vi "Graph_Input_v00.vi"(11 "Control":T7={"PII In 1"={"Lock"=FALSE, "Hold"=FALSE, "P Gain"=0, "P BS"=-5, "I Gain"=0, "I BS"=-10, "I2 G"=0, "I2 BS"=-26, "Scan Amp"=0, "Scan Off"=0, "Scan FS"=0, "SFS BS"=0, "I Max value"=10000, "I2 Max value"=10000, "Scope.Offset"=0, "Trigger Direction"=enum."either", "Scan-PII thresh"=0}, "PII In 2"={"Lock"=FALSE, "Hold"=FALSE, "P Gain"=0, "P BS"=-10, "I Gain"=0, "I BS"=-10, "I2 G"=0, "I2 BS"=-26, "Scan Amp"=0, "Scan Off"=0, "Scan FS"=0, "SFS BS"=0, "I Max value"=10000, "I2 Max value"=10000, "Scope.Offset"=0, "Trigger Direction"=enum."either", "Scan-PII thresh"=0}, "PII In 3"={"Lock"=FALSE, "Hold"=FALSE, "P Gain"=0, "P BS"=-10, "I Gain"=0, "I BS"=-10, "I2 G"=0, "I2 BS"=-26, "Scan Amp"=0, "Scan Off"=0, "Scan FS"=0, "SFS BS"=0, "I Max value"=10000, "I2 Max value"=10000, "Scope.Offset"=0, "Trigger Direction"=enum."either", "Scan-PII thresh"=0}, "PII In 4"={"Lock"=FALSE, "Hold"=FALSE, "P Gain"=0, "P BS"=-10, "I Gain"=0, "I BS"=-10, "I2 G"=0, "I2 BS"=-26, "Scan Amp"=0, "Scan Off"=0, "Scan FS"=0, "SFS BS"=0, "I Max value"=10000, "I2 Max value"=10000, "Scope.Offset"=0, "Trigger Direction"=enum."either", "Scan-PII thresh"=0}, "PII In 5"={"Lock"=FALSE, "Hold"=FALSE, "P Gain"=10, "P BS"=-10, "I Gain"=0, "I BS"=0, "I2 G"=0, "I2 BS"=-26, "Scan Amp"=0, "Scan Off"=0, "Scan FS"=0, "SFS BS"=0, "I Max value"=10000, "I2 Max value"=10000, "Scope.Offset"=0, "Trigger Direction"=enum."either", "Scan-PII thresh"=0}, "PII In 6"={"Lock"=FALSE, "Hold"=FALSE, "P Gain"=0, "P BS"=-10, "I Gain"=0, "I BS"=-10, "I2 G"=0, "I2 BS"=-26, "Scan Amp"=0, "Scan Off"=0, "Scan FS"=0, "SFS BS"=0, "I Max value"=10000, "I2 Max value"=10000, "Scope.Offset"=0, "Trigger Direction"=enum."either", "Scan-PII thresh"=0}, "Error scale"={"Pre-Offset"={"Pre-Offset 1"=2, "Pre-Offset 2"=0, "Pre-Offset 3"=0, "Pre-Offset 4"=0, "Pre-Offset 5"=2, "Pre-Offset 6"=0, "Pre-Offset 7"=0, "Pre-Offset 8"=0}, "Post-Offset "={"Offset 1"=0, "Offset 2"=300, "Offset 3"=0, "Offset 4"=0, "Offset 5"=0, "Offset 6"=0, "Offset 7"=0, "Offset 8"=0}, "Gains"={"Gain 1"=0, "Gain 2"=300, "Gain 3"=0, "Gain 4"=0, "Gain 5"=0, "Gain 6"=0, "Gain 7"=0, "Gain 8"=0}, "Bit Shifts"={"Bit Shift 1"=0, "Bit Shift 2"=300, "Bit Shift 3"=0, "Bit Shift 4"=0, "Bit Shift 5"=0, "Bit Shift 6"=0, "Bit Shift 7"=0, "Bit Shift 8"=0}}, "Lock Thresh"={"Pump A"=2, "Pump B"=0, "EPR"=0, "Graph"=0, "HD A"=0, "HD B"=-10}, "Re-Scan Thresh"={"Pump A"=2, "Pump B"=0, "EPR"=0, "Graph"=-10, "HD A"=0, "HD B"=-10}, "Theta"={"HD A Sin Theta"=2, "HD A Cos Theta"=0, "HD B Sin Theta"=40, "HD B Cos Theta"=0}, "Safety First"={"lim reset"=FALSE, "no limit"=FALSE, "pos slew rate * dt"=0, "neg slew rate * dt"=0, "Hold All"=FALSE, "Count(Ticks)"=0}}) -> (3 "Signals":T3={"PII In 1"={"Lock"=FALSE, "Hold"=FALSE, "P Gain"=0, "P BS"=0, "I Gain"=0, "I BS"=-10, "I2 G"=0, "I2 BS"=-26, "Scan Amp"=0, "Scan Off"=0, "Scan FS"=0, "SFS BS"=0, "I Max value"=10000, "I2 Max value"=10000, "Scope.Offset"=0, "Trigger Direction"=enum."either", "Scan-PII thresh"=0}, "PII In 2"={"Lock"=FALSE, "Hold"=FALSE, "P Gain"=0, "P BS"=0, "I Gain"=0, "I BS"=-10, "I2 G"=0, "I2 BS"=-26, "Scan Amp"=0, "Scan Off"=0, "Scan FS"=0, "SFS BS"=0, "I Max value"=10000, "I2 Max value"=10000, "Scope.Offset"=0, "Trigger Direction"=enum."either", "Scan-PII thresh"=0}, "PII In 3"={"Lock"=FALSE, "Hold"=FALSE, "P Gain"=0, "P BS"=0, "I Gain"=0, "I BS"=-10, "I2 G"=0, "I2 BS"=-26, "Scan Amp"=0, "Scan Off"=0, "Scan FS"=0, "SFS BS"=0, "I Max value"=10000, "I2 Max value"=10000, "Scope.Offset"=0, "Trigger Direction"=enum."either", "Scan-PII thresh"=0}, "PII In 4"={"Lock"=FALSE, "Hold"=FALSE, "P Gain"=0, "P BS"=0, "I Gain"=0, "I BS"=-10, "I2 G"=0, "I2 BS"=-26, "Scan Amp"=0, "Scan Off"=0, "Scan FS"=0, "SFS BS"=0, "I Max value"=10000, "I2 Max value"=10000, "Scope.Offset"=0, "Trigger Direction"=enum."either", "Scan-PII thresh"=0}, "PII In 5"={"Lock"=FALSE, "Hold"=FALSE, "P Gain"=0, "P BS"=-5, "I Gain"=0, "I BS"=-10, "I2 G"=0, "I2 BS"=-26, "Scan Amp"=0, "Scan Off"=0, "Scan FS"=0, "SFS BS"=0, "I Max value"=10000, "I2 Max value"=10000, "Scope.Offset"=0, "Trigger Direction"=enum."either", "Scan-PII thresh"=0}, "PII In 6"={"Lock"=FALSE, "Hold"=FALSE, "P Gain"=0, "P BS"=-10, "I Gain"=0, "I BS"=-10, "I2 G"=0, "I2 BS"=-26, "Scan Amp"=0, "Scan Off"=0, "Scan FS"=0, "SFS BS"=0, "I Max value"=10000, "I2 Max value"=10000, "Scope.Offset"=0, "Trigger Direction"=enum."either", "Scan-PII thresh"=0}, "Lock Thresh"={"Pump A"=2, "Pump B"=0, "EPR"=0, "Graph"=-10, "HD A"=0, "HD B"=-10}, "Re-Scan Thresh"={"Pump A"=2, "Pump B"=0, "EPR"=0, "Graph"=-10, "HD A"=0, "HD B"=-10}, "Safety First"={"lim reset"=FALSE, "no limit"=FALSE, "pos slew rate * dt"=10, "neg slew rate * dt"=-10, "Hold All"=FALSE, "Count(Ticks)"=0}, "Graph Errors"={"Pump A"=0, "Pump B"=1800, "EPR"=0, "Graph"=0, "HD A"=0, "HD B"=0}}, 7 "HD Errors xp":T1)   [LabVIEW 2010]
doc: "Reads in and scales 8 inputs from the FPGA. For each homodyne lock 2 orthogonal error signals are combined in order to lock the local oscillator to an arbitrary phase."
uses:
  Strict Type Defs/FPGA Inputs Graph.ctl
  Strict Type Defs/Graph Errors.ctl
  Strict Type Defs/Control Graph Input.ctl
  Strict Type Defs/PII individual.ctl
  Strict Type Defs/Error Scale Graph.ctl
  Strict Type Defs/Lock Thresh Graph.ctl
  Strict Type Defs/Theta graph.ctl
  Strict Type Defs/Safety First.ctl
  Strict Type Defs/Signals Graph.ctl
  <vilib>/eio/EIONode/EIONode.xnode
  <vilib>/rvi/eio/nirviEIOImplementation/nirviEIOImplementation.xnode
  <vilib>/rvi/eio/common/nirviEmuClasses.ctl
  <vilib>/rvi/eio/common/nirviEmuTemplateMethod_noerrors.vi
panel:
  in  "x p Errors":T1={"HD A x"=0, "HD A p"=1800, "HD B x"=0, "HD B p"=0}
  out "Error Signals":T2={"Pump A"=0, "Pump B"=1800, "EPR"=0, "Graph"=0, "HD A"=0, "HD B"=0}
  in  "Signals":T3={"PII In 1"={"Lock"=FALSE, "Hold"=FALSE, "P Gain"=0, "P BS"=0, "I Gain"=0, "I BS"=-10, "I2 G"=0, "I2 BS"=-26, "Scan Amp"=0, "Scan Off"=0, "Scan FS"=0, "SFS BS"=0, "I Max value"=10000, "I2 Max value"=10000, "Scope.Offset"=0, "Trigger Direction"=enum."either", "Scan-PII thresh"=0}, "PII In 2"={"Lock"=FALSE, "Hold"=FALSE, "P Gain"=0, "P BS"=0, "I Gain"=0, "I BS"=-10, "I2 G"=0, "I2 BS"=-26, "Scan Amp"=0, "Scan Off"=0, "Scan FS"=0, "SFS BS"=0, "I Max value"=10000, "I2 Max value"=10000, "Scope.Offset"=0, "Trigger Direction"=enum."either", "Scan-PII thresh"=0}, "PII In 3"={"Lock"=FALSE, "Hold"=FALSE, "P Gain"=0, "P BS"=0, "I Gain"=0, "I BS"=-10, "I2 G"=0, "I2 BS"=-26, "Scan Amp"=0, "Scan Off"=0, "Scan FS"=0, "SFS BS"=0, "I Max value"=10000, "I2 Max value"=10000, "Scope.Offset"=0, "Trigger Direction"=enum."either", "Scan-PII thresh"=0}, "PII In 4"={"Lock"=FALSE, "Hold"=FALSE, "P Gain"=0, "P BS"=0, "I Gain"=0, "I BS"=-10, "I2 G"=0, "I2 BS"=-26, "Scan Amp"=0, "Scan Off"=0, "Scan FS"=0, "SFS BS"=0, "I Max value"=10000, "I2 Max value"=10000, "Scope.Offset"=0, "Trigger Direction"=enum."either", "Scan-PII thresh"=0}, "PII In 5"={"Lock"=FALSE, "Hold"=FALSE, "P Gain"=0, "P BS"=-5, "I Gain"=0, "I BS"=-10, "I2 G"=0, "I2 BS"=-26, "Scan Amp"=0, "Scan Off"=0, "Scan FS"=0, "SFS BS"=0, "I Max value"=10000, "I2 Max value"=10000, "Scope.Offset"=0, "Trigger Direction"=enum."either", "Scan-PII thresh"=0}, "PII In 6"={"Lock"=FALSE, "Hold"=FALSE, "P Gain"=0, "P BS"=-10, "I Gain"=0, "I BS"=-10, "I2 G"=0, "I2 BS"=-26, "Scan Amp"=0, "Scan Off"=0, "Scan FS"=0, "SFS BS"=0, "I Max value"=10000, "I2 Max value"=10000, "Scope.Offset"=0, "Trigger Direction"=enum."either", "Scan-PII thresh"=0}, "Lock Thresh"={"Pump A"=2, "Pump B"=0, "EPR"=0, "Graph"=-10, "HD A"=0, "HD B"=-10}, "Re-Scan Thresh"={"Pump A"=2, "Pump B"=0, "EPR"=0, "Graph"=-10, "HD A"=0, "HD B"=-10}, "Safety First"={"lim reset"=FALSE, "no limit"=FALSE, "pos slew rate * dt"=10, "neg slew rate * dt"=-10, "Hold All"=FALSE, "Count(Ticks)"=0}, "Graph Errors"={"Pump A"=0, "Pump B"=1800, "EPR"=0, "Graph"=0, "HD A"=0, "HD B"=0}}
  in  "Error Signals":T2
  in  "FPGA Inputs":T10
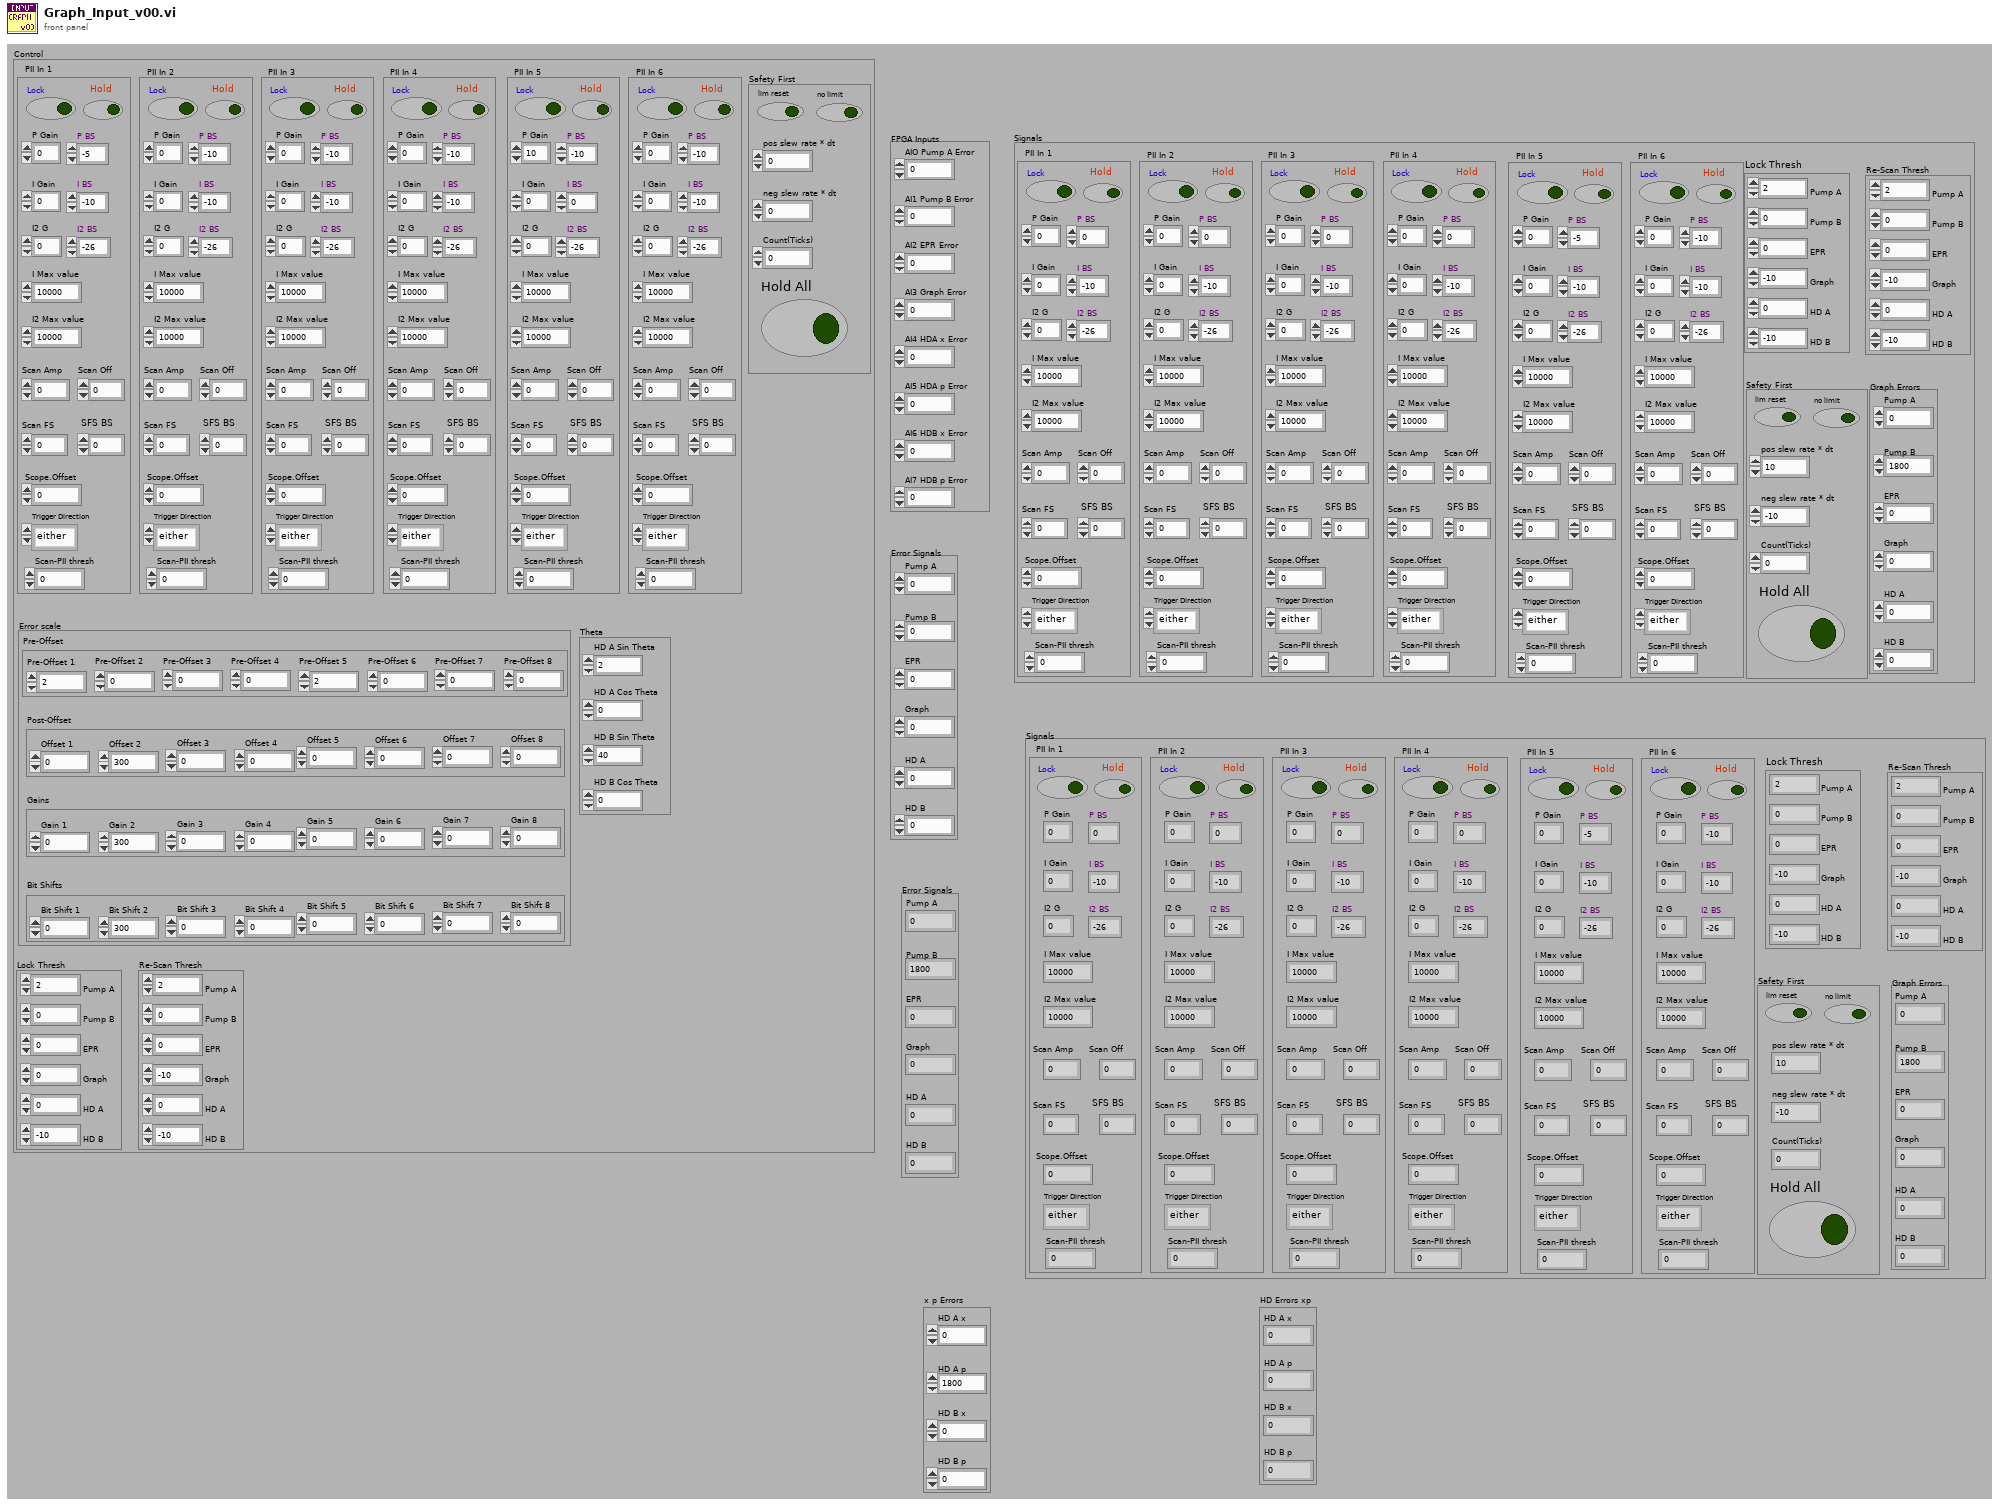
[diagram p1: front panel]
types:
  T1 = cluster{"HD A x":i16, "HD A p":i16, "HD B x":i16, "HD B p":i16}
  T2 = typedef "Graph Errors.ctl" = cluster{"Pump A":i16, "Pump B":i16, "EPR":i16, "Graph":i16, "HD A":i16, "HD B":i16}
  T3 = typedef "Signals Graph.ctl" = cluster{"PII In 1":T4, "PII In 2":T4, "PII In 3":T4, "PII In 4":T4, "PII In 5":T4, "PII In 6":T4, "Lock Thresh":T5, "Re-Scan Thresh":T5, "Safety First":T6, "Graph Errors":T2}
  T4 = typedef "PII individual.ctl" = cluster{"Lock":bool, "Hold":bool, "P Gain":i32, "P BS":i16, "I Gain":i32, "I BS":i16, "I2 G":i32, "I2 BS":i16, "Scan Amp":i16, "Scan Off":i16, "Scan FS":u16, "SFS BS":i16, "I Max value":i32, "I2 Max value":i32, "Scope.Offset":i16, "Trigger Direction":enum8{"either", "minus-plus", "plus-minus"}, "Scan-PII thresh":i16}
  T5 = typedef "Lock Thresh Graph.ctl" = cluster{"Pump A":i16, "Pump B":i16, "EPR":i16, "Graph":i16, "HD A":i16, "HD B":i16}
  T6 = typedef "Safety First.ctl" = cluster{"lim reset":bool, "no limit":bool, "pos slew rate * dt":i16, "neg slew rate * dt":i16, "Hold All":bool, "Count(Ticks)":u32}
  T7 = typedef "Control Graph Input.ctl" = cluster{"PII In 1":T4, "PII In 2":T4, "PII In 3":T4, "PII In 4":T4, "PII In 5":T4, "PII In 6":T4, "Error scale":T8, "Lock Thresh":T5, "Re-Scan Thresh":T5, "Theta":T9, "Safety First":T6}
  T8 = typedef "Error Scale Graph.ctl" = cluster{"Pre-Offset":cluster{"Pre-Offset 1":i16, "Pre-Offset 2":i16, "Pre-Offset 3":i16, "Pre-Offset 4":i16, "Pre-Offset 5":i16, "Pre-Offset 6":i16, "Pre-Offset 7":i16, "Pre-Offset 8":i16}, "Post-Offset ":cluster{"Offset 1":i16, "Offset 2":i16, "Offset 3":i16, "Offset 4":i16, "Offset 5":i16, "Offset 6":i16, "Offset 7":i16, "Offset 8":i16}, "Gains":cluster{"Gain 1":i16, "Gain 2":i16, "Gain 3":i16, "Gain 4":i16, "Gain 5":i16, "Gain 6":i16, "Gain 7":i16, "Gain 8":i16}, "Bit Shifts":cluster{"Bit Shift 1":i16, "Bit Shift 2":i16, "Bit Shift 3":i16, "Bit Shift 4":i16, "Bit Shift 5":i16, "Bit Shift 6":i16, "Bit Shift 7":i16, "Bit Shift 8":i16}}
  T9 = typedef "Theta graph.ctl" = cluster{"HD A Sin Theta":i32, "HD A Cos Theta":i32, "HD B Sin Theta":i32, "HD B Cos Theta":i32}
  T10 = typedef "FPGA Inputs Graph.ctl" = cluster{"AIO Pump A Error":i16, "AI1 Pump B Error":i16, "AI2 EPR Error":i16, "AI3 Graph Error":i16, "AI4 HDA x Error":i16, "AI5 HDA p Error":i16, "AI6 HDB x Error":i16, "AI7 HDB p Error":i16}
  T11 = cluster{"Offset 1":i16, "Offset 2":i16, "Offset 3":i16, "Offset 4":i16, "Offset 5":i16, "Offset 6":i16, "Offset 7":i16, "Offset 8":i16}
  T12 = cluster{"Bit Shift 1":i16, "Bit Shift 2":i16, "Bit Shift 3":i16, "Bit Shift 4":i16, "Bit Shift 5":i16, "Bit Shift 6":i16, "Bit Shift 7":i16, "Bit Shift 8":i16}
  T13 = cluster{"Gain 1":i16, "Gain 2":i16, "Gain 3":i16, "Gain 4":i16, "Gain 5":i16, "Gain 6":i16, "Gain 7":i16, "Gain 8":i16}
  T14 = cluster{"Pre-Offset 1":i16, "Pre-Offset 2":i16, "Pre-Offset 3":i16, "Pre-Offset 4":i16, "Pre-Offset 5":i16, "Pre-Offset 6":i16, "Pre-Offset 7":i16, "Pre-Offset 8":i16}
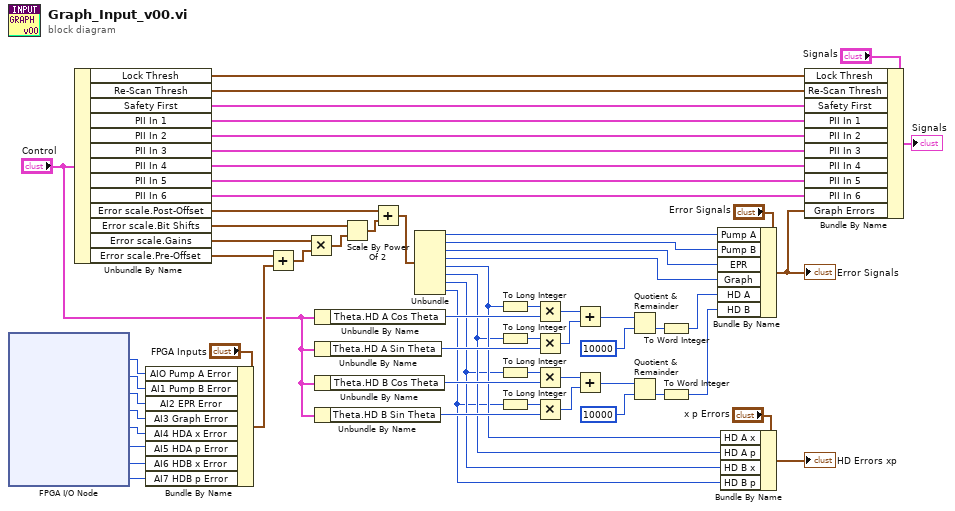
[diagram p0: block diagram]
diagram:
  n1 = xnode "FPGA I/O Node"() -> ("Connector0/AI0"=w1:i16, "Connector0/AI1"=w56:i16, "Connector0/AI2"=w55:i16, "Connector0/AI3"=w54:i16, "Connector0/AI4"=w53:i16, "Connector0/AI5"=w52:i16, "Connector0/AI6"=w57:i16, "Connector0/AI7"=w58:i16)  [unwired: 8 in, 8 out]
  n2 = Unbundle By Name("Control") -> ("Lock Thresh"=w17:T5, "Re-Scan Thresh"=w16:T5, "Safety First"=w18:T6, "PII In 1"=w43:T4, "PII In 2"=w42:T4, "PII In 3"=w41:T4, "PII In 4"=w40:T4, "PII In 5"=w21:T4, "PII In 6"=w20:T4, "Error scale.Post-Offset"=w62:T11, "Error scale.Bit Shifts"=w3:T12, "Error scale.Gains"=w59:T13, "Error scale.Pre-Offset"=w60:T14)
  n3 = Bundle By Name(cluster="FPGA Inputs", "AIO Pump A Error"=w1, "AI1 Pump B Error"=w56, "AI2 EPR Error"=w55, "AI3 Graph Error"=w54, "AI4 HDA x Error"=w53, "AI5 HDA p Error"=w52, "AI6 HDB x Error"=w57, "AI7 HDB p Error"=w58) -> (w39:T10)
  n4 = Add(x=w60, y=w39) -> (x+y=w61:T10)
  n5 = Multiply(x=w59, y=w61) -> (x*y=w5:T10)
  n6 = Unbundle By Name("Control") -> ("Theta.HD A Cos Theta"=w36:i32)
  n7 = Unbundle By Name("Control") -> ("Theta.HD A Sin Theta"=w32:i32)
  n8 = Unbundle By Name("Control") -> ("Theta.HD B Cos Theta"=w25:i32)
  n9 = Unbundle By Name("Control") -> ("Theta.HD B Sin Theta"=w29:i32)
  n10 = Scale By Power Of 2(n=w3, x=w5) -> (x*2^n=w4:T10)
  n11 = Add(x=w62, y=w4) -> (x+y=w2:T10)
  n12 = Unbundle(w2) -> ("AIO Pump A Error"=w49:i16, "AI1 Pump B Error"=w48:i16, "AI2 EPR Error"=w47:i16, "AI3 Graph Error"=w46:i16, "AI4 HDA x Error"=w10:i16, "AI5 HDA p Error"=w9:i16, "AI6 HDB x Error"=w8:i16, "AI7 HDB p Error"=w7:i16)
  n13 = To Long Integer(number=w10) -> (32bit integer=w37:i32)
  n14 = To Long Integer(number=w9) -> (32bit integer=w33:i32)
  n15 = To Long Integer(number=w8) -> (32bit integer=w24:i32)
  n16 = To Long Integer(number=w7) -> (32bit integer=w28:i32)
  n17 = Multiply(x=w37, y=w36) -> (x*y=w35:i32)
  n18 = Multiply(x=w33, y=w32) -> (x*y=w31:i32)
  n19 = Multiply(x=w24, y=w25) -> (x*y=w26:i32)
  n20 = Multiply(x=w28, y=w29) -> (x*y=w30:i32)
  n21 = Add(x=w35, y=w31) -> (x+y=w34:i32)
  n22 = Add(x=w26, y=w30) -> (x+y=w27:i32)
  n23 = Quotient & Remainder(x=w34, y=10000) -> (floor(x/y)=w13:i32)  [unwired: 1 out]
  n24 = Quotient & Remainder(x=w27, y=10000) -> (floor(x/y)=w15:i32)  [unwired: 1 out]
  n25 = To Word Integer(number=w13) -> (16bit integer=w12:i16)
  n26 = To Word Integer(number=w15) -> (16bit integer=w14:i16)
  n27 = Bundle By Name(cluster="Error Signals", "Pump A"=w49, "Pump B"=w48, "EPR"=w47, "Graph"=w46, "HD A"=w12, "HD B"=w14) -> (w19:T2)
  "Error Signals" <- w19
  n28 = Bundle By Name(cluster="x p Errors", "HD A x"=w10, "HD A p"=w9, "HD B x"=w8, "HD B p"=w7) -> (→"HD Errors xp":T1)
  n29 = Bundle By Name(cluster="Signals", "Lock Thresh"=w17, "Re-Scan Thresh"=w16, "Safety First"=w18, "PII In 1"=w43, "PII In 2"=w42, "PII In 3"=w41, "PII In 4"=w40, "PII In 5"=w21, "PII In 6"=w20, "Graph Errors"=w19) -> (→"Signals":T3)
